vi "Get-browse-dialog-pattern.vi"(8 "error in (no error)":errorcluster, 11 "SettingsFile in":refnum<class "SettingsFile.lvclass">) -> (0 "error out":errorcluster, 1 "Pattern label":string, 2 "Pattern":string, 3 "SettingsFile out":refnum<class "SettingsFile.lvclass">)   [LabVIEW 2013, in "SettingsFile.lvlib" / "SettingsFile.lvclass"]
uses:
  SettingsFile.lvclass
  SettingsFile.lvclass/SettingsFile.ctl
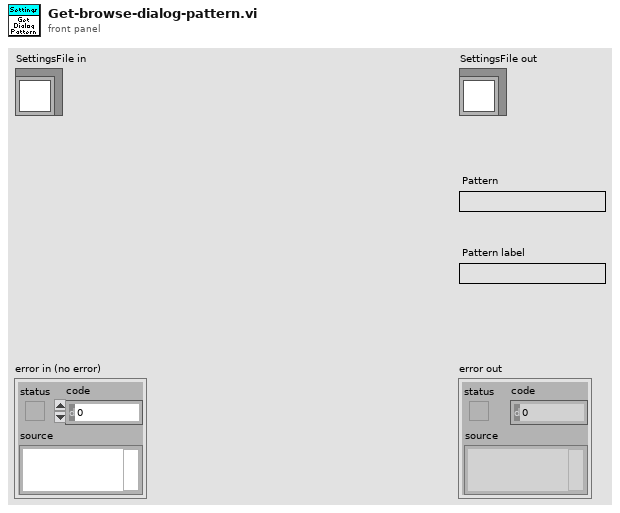
[diagram p1: front panel]
types:
  T1 = enum16{"Not implemented", "Command not recognized", "Invalid input", "No connection", "Timeout", "Invalid file type"}
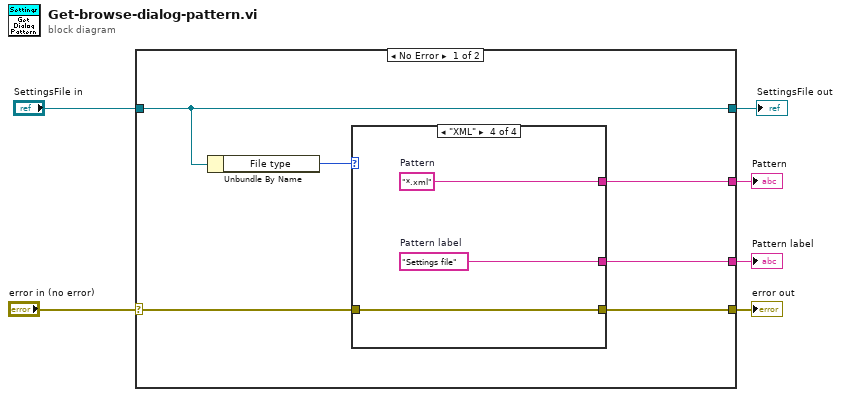
[diagram p0: block diagram]
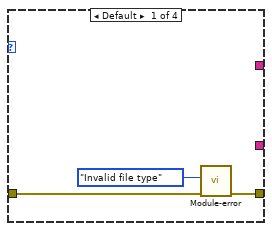
[diagram p2: hidden frame]
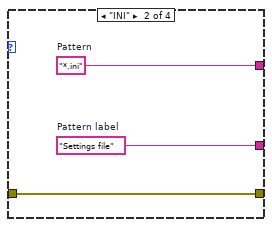
[diagram p3: hidden frame]
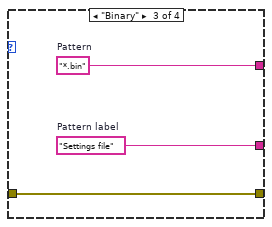
[diagram p4: hidden frame]
diagram:
  n1 = case shown="No Error" "error in (no error)" {
    selector: "error in (no error)" -> [w9 w26]
    tunnel: [w8 w26] -> w5
    tunnel: [w12 w25] -> w3
    tunnel: "SettingsFile in" -> [w12 w25]
    tunnel: [w10 _] -> w2
    tunnel: [w7 _] -> w1
    frame No Error {
      n2 = Unbundle By Name(w12) -> ("File type"=w11:enum16{"XML", "INI", "Binary"})
      n3 = case shown="\"XML\"" w11 {
        tunnel: [_ w18 w21 w24] -> w10
        tunnel: w9 -> [w13 w17 w20 w23]
        tunnel: [w15 w17 w20 w23] -> w8
        tunnel: [_ w16 w19 w22] -> w7
        frame Default {
          n4 = call "Module-error.vi"("error in (no error)"=w13, "Error"=T1."Invalid file type") -> ("error out"=w15:errorcluster)  [unwired: 9 in]
        }
        frame "INI" {
          w16 = "Settings file"  # Pattern label
          w18 = "*.ini"  # Pattern
        }
        frame "Binary" {
          w19 = "Settings file"  # Pattern label
          w21 = "*.bin"  # Pattern
        }
        frame "XML" {
          w22 = "Settings file"  # Pattern label
          w24 = "*.xml"  # Pattern
        }
      }
    }
    frame Error {
    }
  }
  "error out" <- w5
  "SettingsFile out" <- w3
  "Pattern" <- w2
  "Pattern label" <- w1
